vi "App Uninit.vi"(8 "error in (no error)":errorcluster, 10 "Core APIs":T1, 11 "DemoApp in":refnum<class "DemoApp.lvclass">) -> (0 "error out":errorcluster)   [LabVIEW 2020, in "VolatusDemo.lvlib" / "DemoApp.lvclass"]
uses:
  DemoApp.lvclass
  Volatus/Core APIs.ctl
  Volatus/VolatusAPI/VolatusAPI.lvclass
  DemoApp.lvclass/DemoApp.ctl
  Volatus/Volatus.lvlib
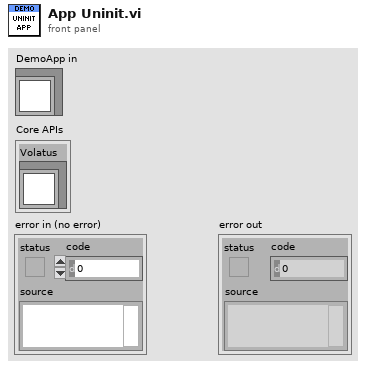
[diagram p1: front panel]
types:
  T1 = typedef "Volatus.lvlib/Core APIs.ctl" = cluster{"Volatus":refnum<class "VolatusAPI.lvclass">}
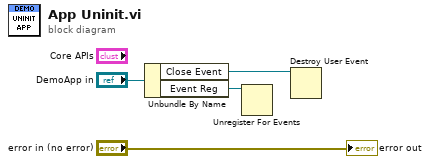
[diagram p0: block diagram]
diagram:
  n1 = Unbundle By Name("DemoApp in") -> ("Close Event"=w1:refnum<user-event>, "Event Reg"=w2:refnum<event-registration>)
  n2 = Unregister For Events(event registration refnum=w2) -> ()  [unwired: 1 in, 1 out]
  n3 = Destroy User Event(user event=w1) -> ()  [unwired: 1 in, 1 out]
  "error out" <- "error in (no error)"
